vi "GetDataFromTable.vi"(0 "DataRecord":T1={"Entête"="", "Scan list"=[], "NbCourbe"=1, "IndCourbe"=0, "NomDon"=["RTêta;", "X&Y;"], "Session "=0, "Date"="", "Time"="", "VarParams"=[], "UserName"="", "ScanTableSize"=[], "VarPar list"=[], "DescKeyword"=""} caption="ScanParams", 1 "XVarParIndex":i32, 3 "ScanlistIndex":i32, 5 "FilesColName":string[](array[string]), 9 "AllDataIn":dbl[][](array[numeric]) format="%#.8f", 11 "error in":errorcluster, 12 "YVarParIndex":i32) -> (2 "Y_VarPar":string, 4 "CurveName":string, 6 "VarPar":string, 8 "X Array":dbl[](array[numeric]), 10 "2D_Data":dbl[][](array[numeric]), 13 "Y Array":dbl[](array[numeric]), 14 "Data Array":dbl[](array[numeric]), 15 "error out":errorcluster)   [LabVIEW 2019]
uses:
  Interface Class/ScanParams.ctl
  <userlib>/GenProg/ArrayTo1DString.vi
  Interface Class/Interface.lvclass
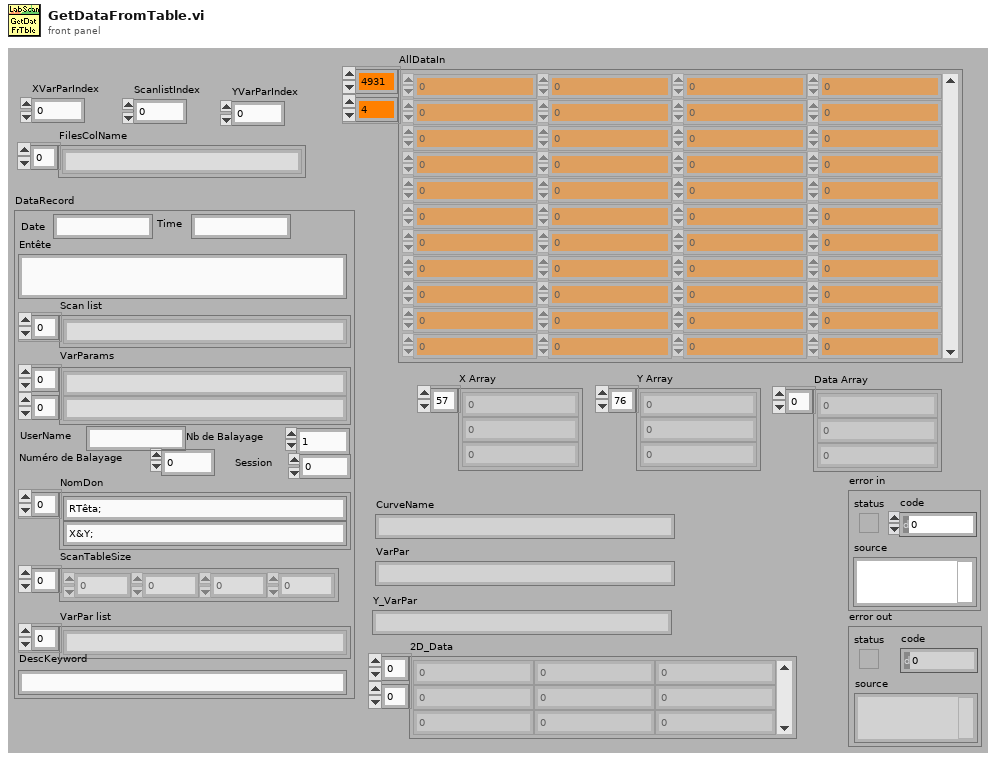
[diagram p1: front panel]
types:
  T1 = typedef "Interface.lvclass/ScanParams.ctl" = cluster{"Entête":string, "Scan list":string[], "NbCourbe":i32, "IndCourbe":i64, "NomDon":string[], "Session ":i32, "Date":string, "Time":string, "VarParams":string[][], "UserName":string, "ScanTableSize":i32[], "VarPar list":string[], "DescKeyword":string}
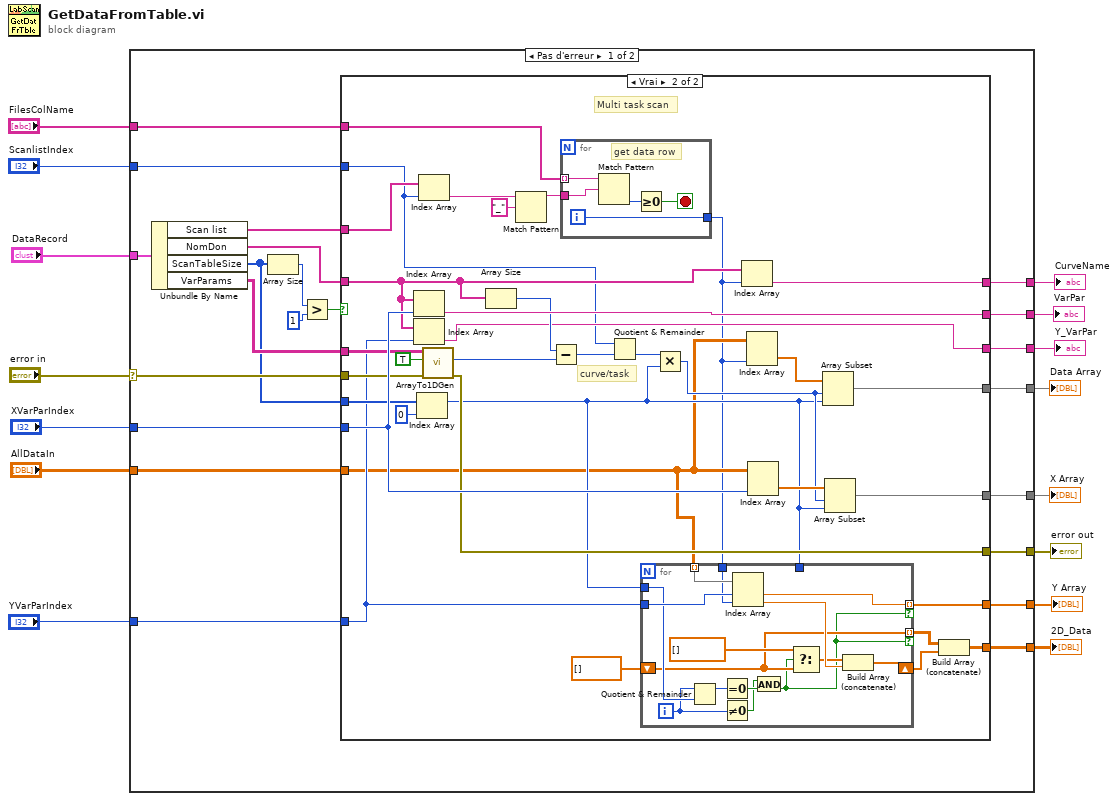
[diagram p0: block diagram]
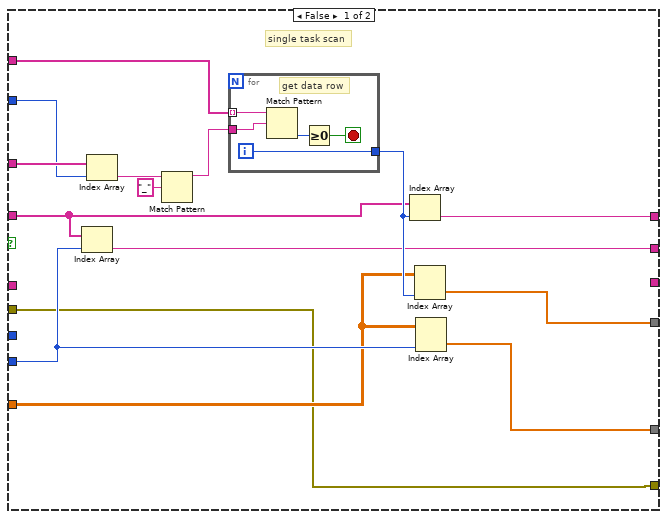
[diagram p2: hidden frame]
diagram:
  n1 = case shown="Pas d'erreur" "error in" {
    selector: "error in" -> [w22 w113]
    tunnel: "ScanlistIndex" -> [w37 _]
    tunnel: "XVarParIndex" -> [w36 _]
    tunnel: "FilesColName" -> [w35 _]
    tunnel: "AllDataIn" -> [w34 _]
    tunnel: "DataRecord" -> [w33 _]
    tunnel: [w27 _] -> w10
    tunnel: [w26 _] -> w9
    tunnel: [w25 _] -> w8
    tunnel: [w24 _] -> w7
    tunnel: [w21 w113] -> w5
    tunnel: [w19 _] -> w4
    tunnel: "YVarParIndex" -> [w18 _]
    tunnel: [w17 _] -> w2
    tunnel: [w16 _] -> w1
    frame No Error {
      n2 = Unbundle By Name(w33) -> ("Scan list"=w32:string[], "NomDon"=w31:string[], "ScanTableSize"=w20:i32[], "VarParams"=w23:string[][])
      n3 = Array Size(array=w20) -> (size(s)=w28:i32)
      n4 = Greater?(x=w28, y=1) -> (0:w29:bool)
      n5 = case shown="Vrai" w29 {
        tunnel: w32 -> [w48 w80]
        tunnel: w37 -> [w47 w62]
        tunnel: w36 -> [w46 w89]
        tunnel: w35 -> [w45 w88]
        tunnel: w34 -> [w44 w63]
        tunnel: w31 -> [w43 w68]
        tunnel: w20 -> [_ w72]
        tunnel: [w41 w76] -> w27
        tunnel: [w40 w74] -> w26
        tunnel: [w39 w86] -> w25
        tunnel: [w42 w87] -> w24
        tunnel: w23 -> [_ w85]
        tunnel: w22 -> [w38 w84]
        tunnel: [w38 w71] -> w21
        tunnel: [_ w65] -> w19
        tunnel: w18 -> [_ w69]
        tunnel: [_ w67] -> w17
        tunnel: [_ w59] -> w16
        frame False {
          # "single task scan"
          n6 = Index Array(array=w43, index=w46) -> (element=w42:string)
          n7 = Index Array(array=w48, index=w47) -> (element=w52:string)
          n8 = Match Pattern(string=w52, regular expression="_" ("expression régulière")) -> (before substring=w50:string)  [unwired: 1 in, 3 out]
          n9 = for {
            tunnel: w45 -> [w53] mode=indexing
            tunnel: w50 -> [w57]
            tunnel: [w56] -> w49
            i -> [w56]
            stop <- w54 stop-if-true
            # "get data row"
            n10 = Match Pattern(string=w53, regular expression=w57) -> (offset past match=w55:i32)  [unwired: 1 in, 3 out]
            n11 = Greater Or Equal To 0?(x=w55) -> (x >= 0?=w54:bool)
          }
          n12 = Index Array(array=w43, index=w49) -> (element=w39:string)
          n13 = Index Array(array=w44, index (col)=w49) -> (element=w41:dbl[])  [unwired: 1 in]
          n14 = Index Array(array=w44, index (col)=w46) -> (element=w40:dbl[])  [unwired: 1 in]
        }
        frame True {
          # "curve/task"
          # "Multi task scan"
          n15 = Index Array(array=w68, index=w89) -> (element=w87:string)
          n16 = Index Array(array=w68, index=w69) -> (element=w67:string)
          n17 = Index Array(array=w72, index=0 ("indice")) -> (element=w66:i32)
          n18 = Index Array(array=w80, index=w62) -> (element=w92:string)
          n19 = call-poly <userlib>:"ArrayTo1DGen.vi"("ErrorIn(No Error)"=w84, "DelArrEnd"=TRUE, "tableau"=w85) -> ("sortie d'erreur"=w71:errorcluster, "Size"=w81:i32)  [unwired: 6 in, 1 out]
          n20 = Array Size(array=w68) -> (size(s)=w82:i32)
          n21 = Match Pattern(string=w92, regular expression="_" ("expression régulière")) -> (before substring=w90:string)  [unwired: 1 in, 3 out]
          n22 = Subtract(x=w82, y=w81) -> (x-y=w79:i32)
          n23 = for {
            tunnel: w88 -> [w108] mode=indexing
            tunnel: w90 -> [w112]
            tunnel: [w111] -> w61
            i -> [w111]
            stop <- w109 stop-if-true
            # "get data row"
            n24 = Match Pattern(string=w108, regular expression=w112) -> (offset past match=w110:i32)  [unwired: 1 in, 3 out]
            n25 = Greater Or Equal To 0?(x=w110) -> (x >= 0?=w109:bool)
          }
          n26 = Quotient & Remainder(x=w62, y=w79) -> (floor(x/y)=w77:i32)  [unwired: 1 out]
          n27 = for {
            tunnel: w63 -> [w107] mode=indexing
            tunnel: w66 -> [_]
            tunnel: w69 -> [w106]
            tunnel: [w105] -> w65 mode=indexing if=w94
            tunnel: w66 -> [w104]
            tunnel: w61 -> [w103]
            tunnel: [w96] -> w60 mode=indexing if=w94
            shift-right: [w99] -> w58
            shift-left: dbl[] [] -> [w96]
            i -> [w95]
            n28 = Quotient & Remainder(x=w95, y=w104) -> (x-y*floor(x/y)=w98:i32)  [unwired: 1 out]
            n29 = Equal To 0?(x=w98) -> (x = 0?=w101:bool)
            n30 = Not Equal To 0?(x=w95) -> (x != 0?=w93:bool)
            n31 = Index Array(array=w107, index #1=w106, index #2=w103) -> (element #1=w105:dbl, element #2=w102:dbl)
            n32 = And(x=w93, y=w101) -> (x .and. y?=w94:bool)
            n33 = Select(t=dbl[] [], s=w94, f=w96) -> (s? t:f=w100:dbl[])
            n34 = Build Array (concatenate)(w100, w102) -> (w99:dbl[])
          }
          n35 = Multiply(x=w77, y=w66) -> (x*y=w73:i32)
          n36 = Index Array(array=w68, index=w61) -> (element=w86:string)
          n37 = Index Array(array=w63, index (col)=w61) -> (element=w78:dbl[])  [unwired: 1 in]
          n38 = Index Array(array=w63, index (col)=w89) -> (element=w75:dbl[])  [unwired: 1 in]
          n39 = Array Subset(array=w78, index=w73, length=w66) -> (w76:dbl[])
          n40 = Array Subset(array=w75, index=w73, length=w66) -> (w74:dbl[])
          n41 = Build Array (concatenate)(w60, w58) -> (w59:dbl[][])
        }
      }
    }
    frame Error {
    }
  }
  "error out" <- w5
  "Data Array" <- w10
  "X Array" <- w9
  "VarPar" <- w7
  "CurveName" <- w8
  "Y Array" <- w4
  "2D_Data" <- w1
  "Y_VarPar" <- w2
